vi "Integral x(t) (obs 90).vi"(2 "dt":dbl=1.0 format="%0.2f", 3 "final condition":dbl format="%0.2f", 4 "initial condition":dbl format="%0.2f", 5 "X":dbl[](array[numeric])) -> (0 "error":i32, 1 "Integral X":dbl[](array[numeric]))   [LabVIEW 2020, in "NI_AALPro.lvlib"]
doc: "The Integral x(t) VI was rewritten in LabVIEW 2009. Replace this VI with the Integral x(t) VI from the <B>Functions</B> palette and select Simpson's Rule as the <B>integration method</B>. Be aware that the Integral x(t) VI in LabVIEW 2009 accepts <B>Initial Condition</B> and <B>Final Condition</B> as array-based inputs.\n\nPerforms the discrete integration of the sampled signal <B>X</B>.\n\nIntegral x(t) calculates a definite integral. The value of the output array at any value x is the area under the curve of the input array between 0 and x."
uses:
  <vilib>/Analysis/NI_AALPro.lvlib
  <resource>/lvanlys.dll
panel:
  # "Integral x(t)"
  # "This VI is obsolete !!!\nYou should replace this VI in your diagram with the Integral x(t)\nVI and select Simpson's Rule in the integration method.\n\nNOTE:   If you have wired to the initial condition and \n              final condition inputs of this obsolete VI, \n              please be aware that the new Integral x(t) VI\n              accepts Initial Condition and Finial Condition \n              as array-based inputs."
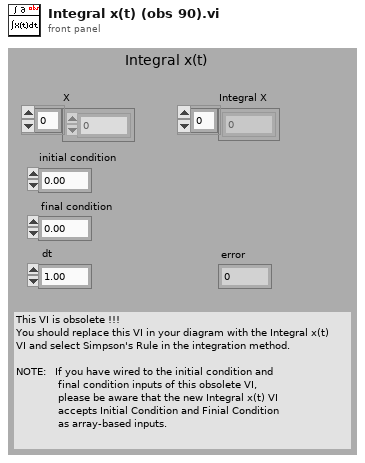
[diagram p1: front panel]
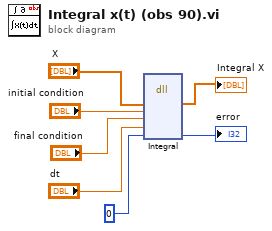
[diagram p0: block diagram]
diagram:
  n1 = dll-call lib="e:/builds/penguin/labview/branches/2020/dev/dist/resource/lvanlys.*" fn="Integral"("X"="X", "initial condition"="initial condition", "final condition"="final condition", "dt"="dt", "error"=0) -> ("X"=→"Integral X":dbl[], "error"=→"error":i32)  [unwired: 6 in, 3 out]
